vi "RT Driver VI.vi"(7 "Operation":T1, 11 "Device Reference in":T2 format="%.0x") -> (0 "Error Code":i32)   [LabVIEW 2026, in "Nominal Core Streaming Engine.lvlib"]
uses:
  Nominal Core Streaming Engine.lvlib
  <vilib>/NI VeriStand/Custom Device API/Custom Device Item Ref.ctl
  <vilib>/NI VeriStand/Custom Device API/Hardware Interface Driver VI Operation.ctl
  Shared/Compiled.Settings.ctl
  Shared/compiled stream data.ctl
  Shared/stream configuration mode.ctl
  Shared/time convert type.ctl
  <vilib>/NI/NIVS Inline Async API/_VS Inline Async API/VS Inline Async API/VS Inline Async API.lvclass
  <vilib>/NI/NIVS Inline Async API/_VS Inline Async API/VS Inline Async API/VS Inline Async API.lvclass/VS Inline Async API.ctl
  <vilib>/NI/NIVS Inline Async API/_Data Access Engine/Data Access Engine/Data Access Engine.lvclass/Data Access Engine.ctl
  <vilib>/NI/NIVS Inline Async API/_Data Access Engine/Access Type Classes/Write/Write.lvclass/Write.ctl
  <vilib>/NI/NIVS Inline Async API/_Data Access Engine/Access Type Classes/ReadWrite/ReadWrite.lvclass/ReadWrite.ctl
  <vilib>/NI/NIVS Inline Async API/_Data Access Engine/Access Type Classes/Read/Read.lvclass/Read.ctl
  <vilib>/NI/NIVS Inline Async API/_Data Access Engine/Data Access Engine/Methods/Data.Engine.Read Data from HW.vi
  <vilib>/NI/NIVS Inline Async API/_VS Inline Async API/Error Handling Process/SubVIs/Error.GetError.vi
  <vilib>/NI/NIVS Inline Async API/_Data Access Engine/Data Access Engine/Methods/Data.Engine.Write Data to HW.vi
  <vilib>/NI/NIVS Inline Async API/_Data Access Engine/Access Type Classes/ReadWrite/ReadWrite.EngineData.vi
  <vilib>/NI/NIVS Inline Async API/_Data Access Engine/Access Type Classes/Write/Write.EngineData.vi
  <vilib>/NI/NIVS Inline Async API/_Data Access Engine/Access Type Classes/Read/Read.EngineData.vi
  <vilib>/NI VeriStand/Custom Device API/NI VeriStand - Get Channel Value by Data Reference.vi
  <vilib>/NI VeriStand/Custom Device API/NI VeriStand - Set Channel Value by Data Reference.vi
  <vilib>/NI VeriStand/Custom Device API/NI VeriStand - Set Channel Values by Block Data Reference.vi
  <vilib>/NI VeriStand/Custom Device API/NI VeriStand - Get Channel Values by Block Data Reference.vi
  Shared/Constants.vi
  Nominal Core Streaming.Async.vi
  <vilib>/NI VeriStand/Custom Device API/Get Item Property (Variant).vi
  <vilib>/NI VeriStand/Custom Device API/Global Data Refs.vi
  <vilib>/NI VeriStand/Custom Device API/Custom Device API.lvlib
  Shared/Nominal Core Streaming Shared.lvlib
  <vilib>/NI VeriStand/Custom Device Tools/Custom Device Utility Library/Custom Device Utility Library.lvlib
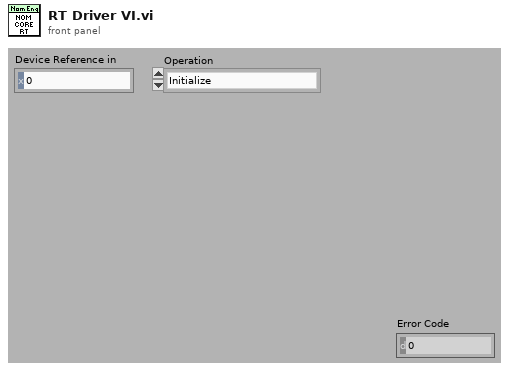
[diagram p1: front panel]
types:
  T1 = typedef "Custom Device API.lvlib/Hardware Interface Driver VI Operation.ctl" = enum16{"Initialize", "Start", "Read Data from HW", "Write Data to HW", "Close"}
  T2 = typedef "Custom Device API.lvlib/Custom Device Item Ref.ctl" = u64
  T3 = cluster{"Async":refnum<class "VS Inline Async API.lvclass">}
  T4 = typedef "Nominal Core Streaming Shared.lvlib/Compiled.Settings.ctl" = cluster{"Name":string, "Async Init Timeout":u16, "stream":T5}
  T5 = typedef "Nominal Core Streaming Shared.lvlib/compiled stream data.ctl" = cluster{"stream name":string, "Base URL":string, "api key":string, "identifier selection":T6, "asset ID":string, "dataset name":string, "dataset ID":string, "associated channels":cluster{"Name":string, "Path":string}[], "fallback avro path":path, "time source":T7, "buffer size":u32}
  T6 = typedef "Nominal Core Streaming Shared.lvlib/stream configuration mode.ctl" = enum16{"Asset Identifier and Dataset Name", "Dataset Identifier"}
  T7 = typedef "Nominal Core Streaming Shared.lvlib/time convert type.ctl" = enum16{"to timestamp", "relative seconds"}
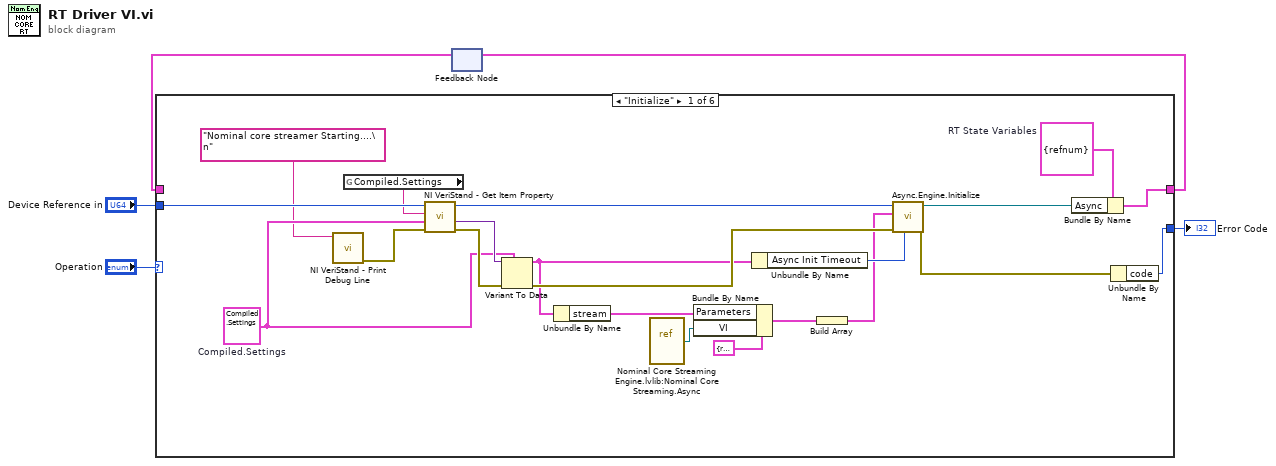
[diagram p0: block diagram]
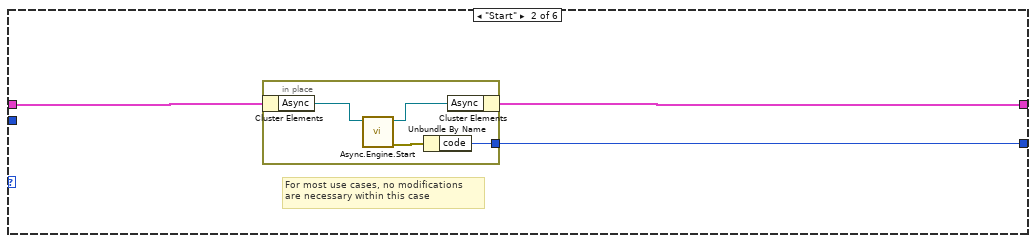
[diagram p2: hidden frame]
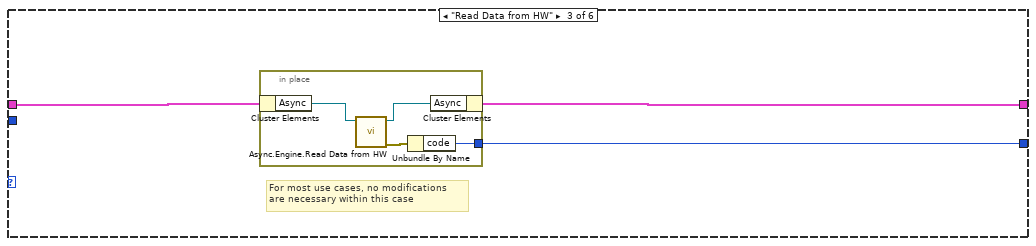
[diagram p3: hidden frame]
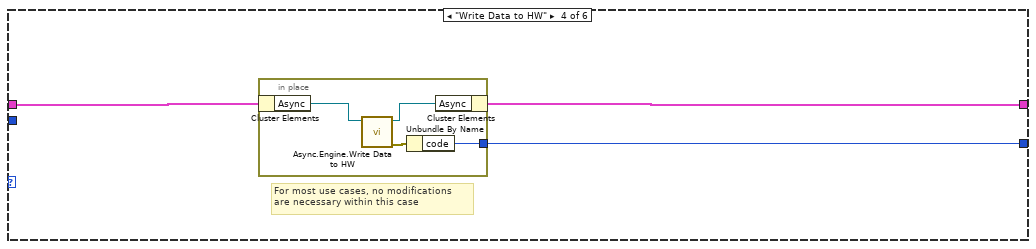
[diagram p4: hidden frame]
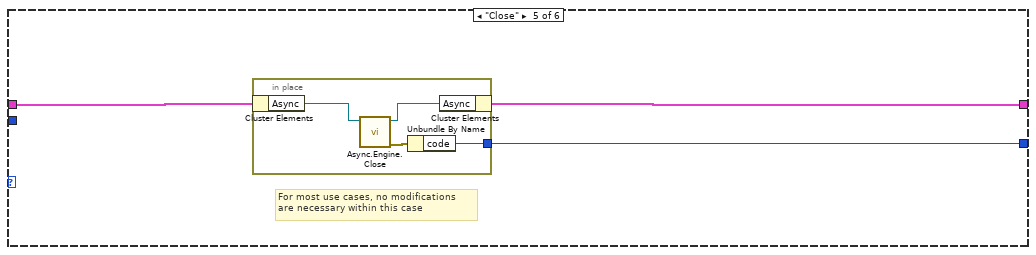
[diagram p5: hidden frame]
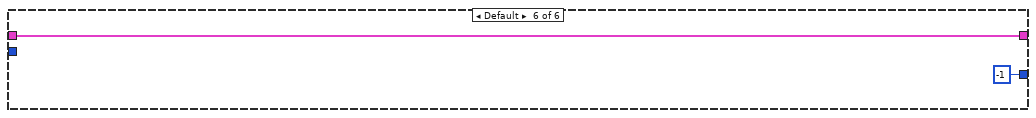
[diagram p6: hidden frame]
diagram:
  n1 = feedback #1() -> (w3:T3)  [unwired: 1 out]
  n2 = case shown="\"Initialize\"" "Operation" {
    tunnel: [w24 w28 w34 w41 w49 w56] -> w4
    tunnel: w3 -> [_ w29 w36 w42 w50 w56]
    tunnel: "Device Reference in" -> [w23 _ _ _ _ _]
    tunnel: [w26 w27 w35 w43 w48 -1 ("code")] -> w1
    frame "Initialize" {
      w18 = T3 {"Async"=refnum}  # RT State Variables
      w19 = T4 {"Name"="", "Async Init Timeout"=0, "stream"={"stream name"="", "Base URL"="https://api.gov.nominal.io/api/", "api key"="", "identifier selection"=enum."Asset Identifier and Dataset Name", "asset ID"="", "dataset name"="", "dataset ID"="", "associated channels"=[], "fallback avro path"=path "", "time source"=enum."to timestamp", "buffer size"=0}}  # Compiled.Settings
      n3 = call <vilib>:"NI VeriStand - Print Debug Line.vi"("Message"="Nominal core streamer Starting....\n") -> ("error out"=w9:errorcluster)  [unwired: 10 in]
      n4 = global read "Constants.vi" "Compiled.Settings"() -> (w20:string)
      n5 = call-poly <vilib>:"NI VeriStand - Get Item Property.vi"("error in (no error)"=w9, "Default Value"=w19, "Property Name"=w20, "Item Ref in"=w23) -> ("error out"=w22:errorcluster, "Value"=w21:variant, "Item Ref out"=w14:T2)  [unwired: 4 in, 1 out]
      n6 = Variant To Data(error in=w22, type=w19, Variant=w21) -> (data=w13:T4, error out=w16:errorcluster)
      n7 = Unbundle By Name(w13) -> ("stream"=w12:T5)
      n8 = vi-ref "Nominal Core Streaming Engine.lvlib:Nominal Core Streaming.Async.vi"() -> (w7:refnum<vi>)
      n9 = Bundle By Name(cluster=cluster{"VI":refnum<vi>, "Parameters":variant} {"VI"=refnum, "Parameters"=variant} ("Process"), "Parameters"=w12, "VI"=w7) -> (w17:cluster{"VI":refnum<vi>, "Parameters":variant})
      n10 = Unbundle By Name(w13) -> ("Async Init Timeout"=w15:u16)
      n11 = Build Array(w17) -> (w11:cluster{"VI":refnum<vi>, "Parameters":variant}[])
      n12 = call <vilib>:"Async.Engine.Initialize.vi"("Timeout (ms) (5000)"=w15, "error in (no error)"=w16, "Processes"=w11, "Custom Device Ref"=w14) -> ("error out"=w6:errorcluster, "Async"=w25:refnum<class "VS Inline Async API.lvclass">)  [unwired: 6 in]
      n13 = Bundle By Name(cluster=w18, "Async"=w25) -> (w24:T3)
      n14 = Unbundle By Name(w6) -> ("code"=w26:i32)
    }
    frame "Start" {
      # "For most use cases, no modifications \nare necessary within this case"
      n15 = in-place {
        in-place-border: [w30] -> w27
        n16 = in-place-cluster #2(w29) -> ("Async"=w33:refnum<class "VS Inline Async API.lvclass">)
        n17 = call <vilib>:"Async.Engine.Start.vi"("VS Inline Async API in"=w33) -> ("error out"=w31:errorcluster, "VS Inline Async API out"=w32:refnum<class "VS Inline Async API.lvclass">)  [unwired: 9 in]
        n18 = Unbundle By Name(w31) -> ("code"=w30:i32)
        n19 = in-place-cluster #2("Async"=w32) -> (w28:T3)
      }
    }
    frame "Read Data from HW" {
      # "For most use cases, no modifications \nare necessary within this case"
      n20 = in-place {
        in-place-border: [w38] -> w35
        n21 = in-place-cluster #3(w36) -> ("Async"=w40:refnum<class "VS Inline Async API.lvclass">)
        n22 = call <vilib>:"Async.Engine.Read Data from HW.vi"("Async in"=w40) -> ("error out"=w37:errorcluster, "Async out"=w39:refnum<class "VS Inline Async API.lvclass">)  [unwired: 9 in]
        n23 = Unbundle By Name(w37) -> ("code"=w38:i32)
        n24 = in-place-cluster #3("Async"=w39) -> (w34:T3)
      }
    }
    frame "Write Data to HW" {
      # "For most use cases, no modifications \nare necessary within this case"
      n25 = in-place {
        in-place-border: [w47] -> w43
        n26 = in-place-cluster #4(w42) -> ("Async"=w45:refnum<class "VS Inline Async API.lvclass">)
        n27 = call <vilib>:"Async.Engine.Write Data to HW.vi"("VS Inline Async API in"=w45) -> ("error out"=w46:errorcluster, "VS Inline Async API out"=w44:refnum<class "VS Inline Async API.lvclass">)  [unwired: 9 in]
        n28 = Unbundle By Name(w46) -> ("code"=w47:i32)
        n29 = in-place-cluster #4("Async"=w44) -> (w41:T3)
      }
    }
    frame "Close" {
      # "For most use cases, no modifications \nare necessary within this case"
      n30 = in-place {
        in-place-border: [w52] -> w48
        n31 = in-place-cluster #5(w50) -> ("Async"=w54:refnum<class "VS Inline Async API.lvclass">)
        n32 = call <vilib>:"Async.Engine.Close.vi"("Async in"=w54) -> ("error out"=w51:errorcluster, "Async out"=w53:refnum<class "VS Inline Async API.lvclass">)  [unwired: 9 in]
        n33 = Unbundle By Name(w51) -> ("code"=w52:i32)
        n34 = in-place-cluster #5("Async"=w53) -> (w49:T3)
      }
    }
    frame Default {
    }
  }
  "Error Code" <- w1
  n35 = feedback-in #1(w4) -> ()
